vi "Get Next.vi"(0 "Conditional in":refnum<class "Case Structure.lvclass">, 1 "Linked List Ref":refnum<data-value>, 5 "Active Unique ID":string, 9 "Active Element Index":i32, 11 "error in (no error)":errorcluster) -> (3 "Linked List Ref out":refnum<data-value>, 4 "Executioner out":refnum<class "Executioner.lvclass">, 6 "Active Unique ID out":string, 8 "Test Executive Ref out":refnum<data-value>, 10 "Active Element Index out":i32, 12 "Found":bool, 13 "Complete":bool, 14 "Stop":bool, 15 "error out":errorcluster)   [LabVIEW 2019, in "Test Executive.lvlib" / "Case Structure.lvclass"]
uses:
  <vilib>/gpm_packages/@cs/test-executive/Source/Test Executive/Case Structure/Case Structure.lvclass
  C:/Program Files/National Instruments/LabVIEW 2019/vi.lib/gpm_packages/@cs/test-executive/Source/Test Executive/Executioner/Executioner.lvclass
  <vilib>/gpm_packages/@cs/test-executive/Source/Test Executive/Executioner/Executioner.lvclass
  <vilib>/gpm_packages/@cs/linked-list/Source/Linked List/ILinkedList/ILinked List.lvclass
  <vilib>/gpm_packages/@cs/test-executive/Source/Test Executive/ITestExecutive/ITest Executive.lvclass
  <vilib>/gpm_packages/@cs/run-time-assertions/Source/Assert/Assert.lvclass
  28516125-fb7c-4ac0-a741-55c0088c8a73.vi
  9cce5d6f-acb7-42fe-8a76-34eb137fd1f1.vi
  ae19bcc6-c34a-426c-aaf2-8c0212fd8e02.vi
  24807a66-3041-465e-b619-213d0f35a6f1.vi
  a9d8a70e-5bac-4ef7-9f0f-e1a86a73ed6e.vi
  7a951b47-5b41-47b6-b8c4-e609ade2915c.vi
  60ecfbe6-bfaf-4739-a238-c250300aa515.vi
  e5c56d01-fc27-46d4-835c-91294360ed0c.vi
  8776d587-be4e-442f-99b1-068521ee802a.vi
  0ed79af9-58b9-4d60-a1f6-ce76f0a075ca.vi
  0de81105-60b3-4a47-8276-928f55148d42.vi
  d8486d1a-e973-4190-8b17-fb3190d4489b.vi
  <vilib>/gpm_packages/@cs/linked-list/Source/Linked List/Linked List Ref/Linked List Ref.lvclass
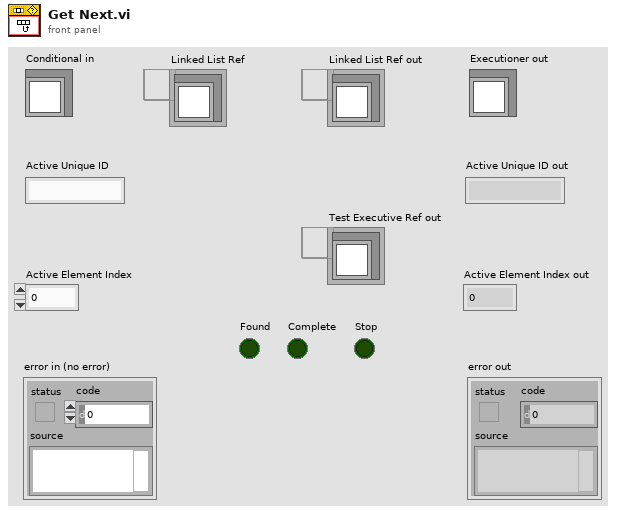
[diagram p1: front panel]
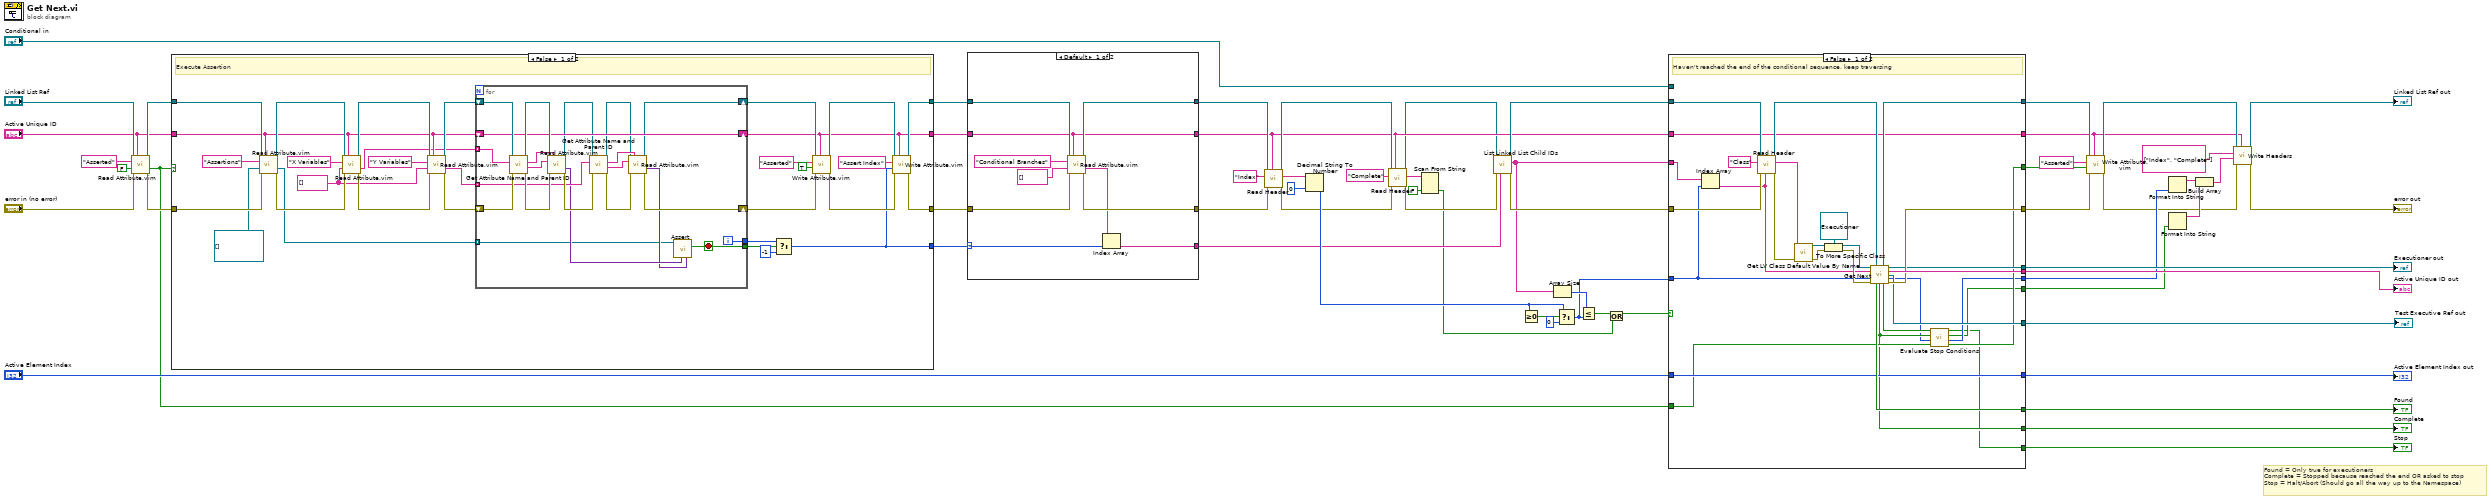
[diagram p0: block diagram]
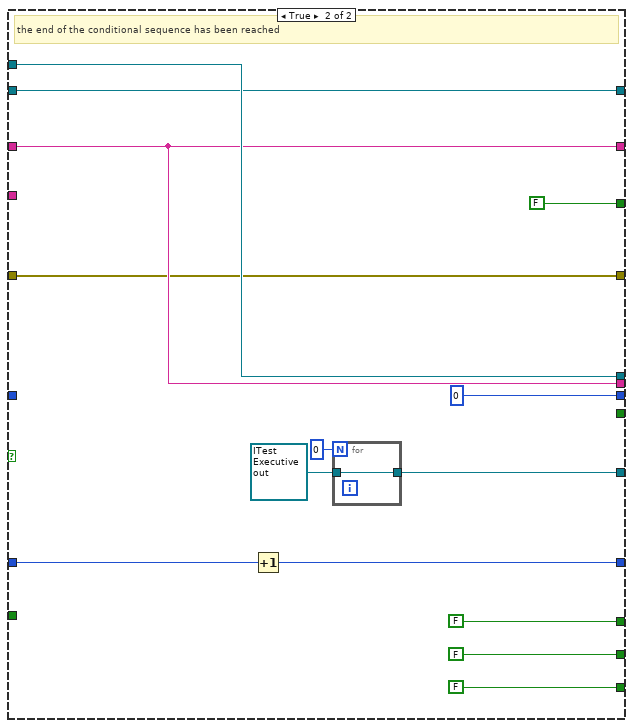
[diagram p2: hidden frame]
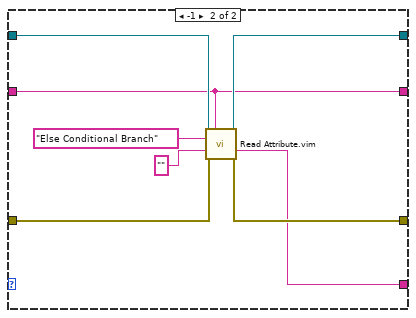
[diagram p3: hidden frame]
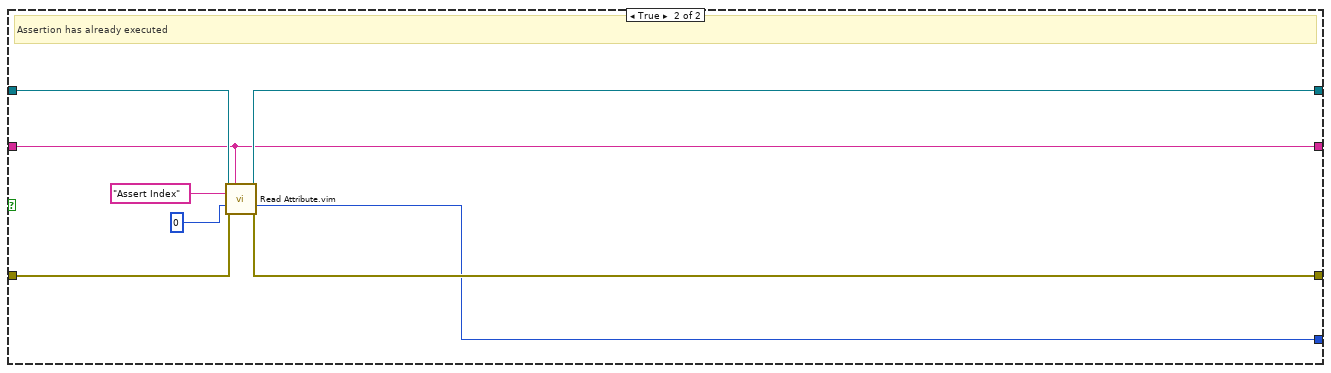
[diagram p4: hidden frame]
diagram:
  # "Found = Only true for executioners\nComplete = Stopped because reached the end OR asked to stop\nStop = Halt/Abort (Should go all the way up to the Namespace)"
  n1 = call "Read Attribute.vim"("Linked List Ref"="Linked List Ref", "Linked List ID"="Active Unique ID", "Attribute Name"="Asserted", "Type"=FALSE, "error in (no error)"="error in (no error)") -> ("Linked List Ref out"=w59:refnum<data-value>, "Attribute"=w1:bool, "error out"=w57:errorcluster)  [unwired: 5 in, 3 out]
  n2 = case shown="False" w1 {
    tunnel: "Active Unique ID" -> [w70 w116]
    tunnel: [w82 w119] -> w24
    tunnel: [w80 w117] -> w26
    tunnel: w59 -> [w87 w120]
    tunnel: w57 -> [w86 w118]
    tunnel: [w66 w116] -> w28
    tunnel: [w62 w115] -> w23
    frame False {
      w75 = string[] []
      # "Execute Assertion"
      n3 = call "Read Attribute.vim"("Linked List Ref"=w87, "Linked List ID"=w70, "Attribute Name"="Assertions", "Type"=refnum<class "Assert.lvclass">[] [] ("Assertions"), "error in (no error)"=w86) -> ("Linked List Ref out"=w91:refnum<data-value>, "Attribute"=w67:refnum<class "Assert.lvclass">[], "error out"=w90:errorcluster)  [unwired: 5 in, 3 out]
      n4 = call "Read Attribute.vim"("Linked List Ref"=w91, "Linked List ID"=w70, "Attribute Name"="X Variables", "Type"=w75, "error in (no error)"=w90) -> ("Linked List Ref out"=w77:refnum<data-value>, "Attribute"=w68:string[], "error out"=w78:errorcluster)  [unwired: 5 in, 3 out]
      n5 = call "Read Attribute.vim"("Linked List Ref"=w77, "Linked List ID"=w70, "Attribute Name"="Y Variables", "Type"=w75, "error in (no error)"=w78) -> ("Linked List Ref out"=w74:refnum<data-value>, "Attribute"=w69:string[], "error out"=w72:errorcluster)  [unwired: 5 in, 3 out]
      n6 = for {
        shift-right: [w99] -> w73
        shift-left: w74 -> [w114]
        shift-right: [w98] -> w71
        shift-left: w72 -> [w112]
        tunnel: w69 -> [w100] mode=indexing
        tunnel: w68 -> [w110] mode=indexing
        tunnel: w67 -> [w93] mode=indexing
        shift-right: [w107] -> w66
        shift-left: w70 -> [w107]
        tunnel: [w97] -> w64
        tunnel: [w96] -> w63
        i -> [w97]
        stop <- w96 stop-if-true
        n7 = call <vilib>:"Get Attribute Name and Parent ID.vi"("error in (no error)"=w112, "Tag"=w110, "Linked List Ref"=w114) -> ("error out"=w111:errorcluster, "Attribute Name"=w109:string, "Linked List ID"=w108:string, "Linked List Ref out"=w113:refnum<data-value>)  [unwired: 5 in]
        n8 = call "Read Attribute.vim"("Linked List Ref"=w113, "Linked List ID"=w108, "Attribute Name"=w109, "error in (no error)"=w111) -> ("Linked List Ref out"=w101:refnum<data-value>, "Attribute"=w95:variant, "error out"=w102:errorcluster)  [unwired: 6 in, 3 out]
        n9 = call <vilib>:"Get Attribute Name and Parent ID.vi"("error in (no error)"=w102, "Tag"=w100, "Linked List Ref"=w101) -> ("error out"=w104:errorcluster, "Attribute Name"=w105:string, "Linked List ID"=w106:string, "Linked List Ref out"=w103:refnum<data-value>)  [unwired: 5 in]
        n10 = call "Read Attribute.vim"("Linked List Ref"=w103, "Linked List ID"=w106, "Attribute Name"=w105, "error in (no error)"=w104) -> ("Linked List Ref out"=w99:refnum<data-value>, "Attribute"=w94:variant, "error out"=w98:errorcluster)  [unwired: 6 in, 3 out]
        n11 = call-dynamic "Assert.vi"("Variable Y"=w94, "Variable X"=w95, "Assert in"=w93) -> ("Assert?"=w96:bool)  [unwired: 8 in]
      }
      n12 = Select(t=w64, s=w63, f=-1) -> (s? t:f=w62:i32)
      n13 = call "Write Attribute.vim"("Linked List ID"=w66, "error in (no error)"=w71, "Attribute"=TRUE, "Attribute Name"="Asserted", "Linked List Ref"=w73) -> ("error out"=w81:errorcluster, "Linked List Ref out"=w83:refnum<data-value>)  [unwired: 3 in, 2 out]
      n14 = call "Write Attribute.vim"("Linked List ID"=w66, "error in (no error)"=w81, "Attribute"=w62, "Attribute Name"="Assert Index", "Linked List Ref"=w83) -> ("error out"=w80:errorcluster, "Linked List Ref out"=w82:refnum<data-value>)  [unwired: 3 in, 2 out]
    }
    frame True {
      # "Assertion has already executed"
      n15 = call "Read Attribute.vim"("Linked List Ref"=w120, "Linked List ID"=w116, "Attribute Name"="Assert Index", "Type"=0, "error in (no error)"=w118) -> ("Linked List Ref out"=w119:refnum<data-value>, "Attribute"=w115:i32, "error out"=w117:errorcluster)  [unwired: 5 in, 3 out]
    }
  }
  n16 = case shown="Default" w23 {
    selector: w23 -> [w125 _]
    tunnel: w28 -> [w123 w133]
    tunnel: [w132 w140] -> w27
    tunnel: w26 -> [w131 w139]
    tunnel: [w130 w138] -> w25
    tunnel: w24 -> [w129 w137]
    tunnel: [w124 w134] -> w22
    tunnel: [w123 w133] -> w14
    frame Default {
      n17 = call "Read Attribute.vim"("Linked List Ref"=w129, "Linked List ID"=w123, "Attribute Name"="Conditional Branches", "Type"=string[] [], "error in (no error)"=w131) -> ("Linked List Ref out"=w130:refnum<data-value>, "Attribute"=w126:string[], "error out"=w132:errorcluster)  [unwired: 5 in, 3 out]
      n18 = Index Array(array=w126, index=w125) -> (element=w124:string)
    }
    frame -1 {
      n19 = call "Read Attribute.vim"("Linked List Ref"=w137, "Linked List ID"=w133, "Attribute Name"="Else Conditional Branch", "Type"="", "error in (no error)"=w139) -> ("Linked List Ref out"=w138:refnum<data-value>, "Attribute"=w134:string, "error out"=w140:errorcluster)  [unwired: 5 in, 3 out]
    }
  }
  n20 = call <vilib>:"Read Header.vi"("Linked List ID"=w14, "error in (no error)"=w27, "Header Name"="Index" ("Attribute Name"), "Linked List Ref"=w25) -> ("error out"=w12:errorcluster, "Header Value"=w34:string, "Linked List Ref out"=w15:refnum<data-value>)  [unwired: 4 in, 1 out]
  n21 = Decimal String To Number(string=w34, default (0L)=0 ("Attribute")) -> (number=w52:i32)  [unwired: 1 in, 1 out]
  n22 = call <vilib>:"Read Header.vi"("Linked List ID"=w14, "error in (no error)"=w12, "Header Name"="Complete" ("Attribute Name"), "Linked List Ref"=w15) -> ("error out"=w11:errorcluster, "Header Value"=w17:string, "Linked List Ref out"=w13:refnum<data-value>)  [unwired: 4 in, 1 out]
  n23 = Scan From String(input string=w17, default 1=FALSE) -> (output 1=w9:bool)  [unwired: 3 in, 3 out]
  n24 = call <vilib>:"List Linked List Child IDs.vi"("Linked List ID"=w22, "error in (no error)"=w11, "Linked List Ref"=w13) -> ("error out"=w50:errorcluster, "Child IDs"=w49:string[], "Linked List Ref out"=w51:refnum<data-value>)  [unwired: 6 in]
  n25 = Greater Or Equal To 0?(x=w52) -> (x >= 0?=w55:bool)
  n26 = Array Size(array=w49) -> (size(s)=w53:i32)
  n27 = Select(t=w52, s=w55, f=0) -> (s? t:f=w48:i32)
  n28 = Less Or Equal?(x=w53, y=w48) -> (x <= y?=w21:bool)
  n29 = Or(x=w21, y=w9) -> (x .or. y?=w10:bool)
  n30 = case shown="False" w10 {
    tunnel: [w160 w173] -> w6
    tunnel: w51 -> [w162 w173]
    tunnel: [w156 w172] -> w4
    tunnel: w50 -> [w164 w172]
    tunnel: w49 -> [w153 _]
    tunnel: w48 -> [w152 _]
    tunnel: [w143 0 ("Active Element Index out")] -> w37
    tunnel: [w149 w181] -> w43
    tunnel: [w159 w177] -> w42
    tunnel: [w158 FALSE ("Found")] -> w47
    tunnel: [w145 FALSE] -> w46
    tunnel: [w141 FALSE] -> w45
    tunnel: "Conditional in" -> [_ w181]
    tunnel: w14 -> [w155 w177]
    tunnel: [w155 w177] -> w2
    tunnel: "Active Element Index" -> [w154 w179]
    tunnel: [w154 w178] -> w40
    tunnel: [w150 w174] -> w29
    tunnel: [w142 _] -> w20
    tunnel: [w147 FALSE] -> w3
    tunnel: w1 -> [w146 _]
    frame False {
      # "Haven't reached the end of the conditional sequence, keep traversing"
      n31 = Index Array(array=w153, index=w152) -> (element=w151:string)
      n32 = call <vilib>:"Read Header.vi"("Linked List ID"=w151, "error in (no error)"=w164, "Header Name"="Class", "Linked List Ref"=w162) -> ("error out"=w157:errorcluster, "Header Value"=w170:string, "Linked List Ref out"=w161:refnum<data-value>)  [unwired: 4 in, 1 out]
      n33 = call <vilib>:"Get LV Class Default Value By Name.vi"("error in (no error)"=w157, "class name"=w170) -> ("error out"=w166:errorcluster, "object"=w169:refnum<class>)  [unwired: 8 in]
      n34 = To More Specific Class(target class=refnum<class "Executioner.lvclass"> refnum ("Test Executive.lvlib:Executioner.lvclass"), reference=w169, error in=w166) -> (specific class reference=w165:refnum<class "Executioner.lvclass">, error out=w167:errorcluster)
      n35 = call-dynamic "Get Next.vi"("Executioner in"=w165, "Linked List Ref"=w161, "Active Unique ID"=w151, "Active Element Index"=w152, "error in (no error)"=w167) -> ("Linked List Ref out"=w160:refnum<data-value>, "Executioner out"=w149:refnum<class "Executioner.lvclass">, "Active Unique ID out"=w159:string, "Test Executive Ref out"=w150:refnum<data-value>, "Active Element Index out"=w144:i32, "Found"=w158:bool, "Complete"=w145:bool, "Stop"=w148:bool, "error out"=w156:errorcluster)  [unwired: 2 in]
      n36 = call <vilib>:"Evaluate Stop Conditions.vi"("Assert"=w146, "Index"=w144, "Complete"=w145, "Stop"=w148) -> ("Asserted"=w147:bool, "Index out"=w143:i32, "Completed"=w142:bool, "Stop out"=w141:bool)  [unwired: 4 in]
    }
    frame True {
      # "the end of the conditional sequence has been reached"
      n37 = Increment(x=w179) -> (x+1=w178:i32)
      n38 = for {
        N: 0 -> [_]
        tunnel: refnum<data-value> refnum ("Test Executive Ref out") -> [w185]
        tunnel: [w185] -> w174
      }
    }
  }
  "Executioner out" <- w43
  "Active Unique ID out" <- w42
  "Active Element Index out" <- w40
  "Found" <- w47
  "Complete" <- w46
  "Stop" <- w45
  "Test Executive Ref out" <- w29
  n39 = call "Write Attribute.vim"("Linked List ID"=w2, "error in (no error)"=w4, "Attribute"=w3, "Attribute Name"="Asserted", "Linked List Ref"=w6) -> ("error out"=w5:errorcluster, "Linked List Ref out"=w7:refnum<data-value>)  [unwired: 3 in, 2 out]
  n40 = Format Into String(w37) -> (resulting string=w31:string)  [unwired: 3 in, 1 out]
  n41 = Format Into String(w20) -> (resulting string=w19:string)  [unwired: 3 in, 1 out]
  n42 = Build Array(w31, w19) -> (w30:string[])
  n43 = call <vilib>:"Write Headers.vi"("Linked List ID"=w2, "error in (no error)"=w5, "Header Values"=w30, "Header Names"=string[] ["Index", "Complete"], "Linked List Ref"=w7) -> ("error out"=→"error out":errorcluster, "Linked List Ref out"=→"Linked List Ref out":refnum<data-value>)  [unwired: 5 in]
